vi "create.algo.watchlist.vi"(11 "Watchlist":T1[](array[typedef]) {"max.bid" format="%.2f"; "min.ask" format="%.2f"}) -> (3 "Memory.Config.Flattened":u64[](array[numeric]) format="%.0x")   [LabVIEW 2020]
uses:
  types/val.algo.pretty.watchlist.ctl
panel:
  out "Memory.Config":u64[][](array[numeric]) format="%.0x"
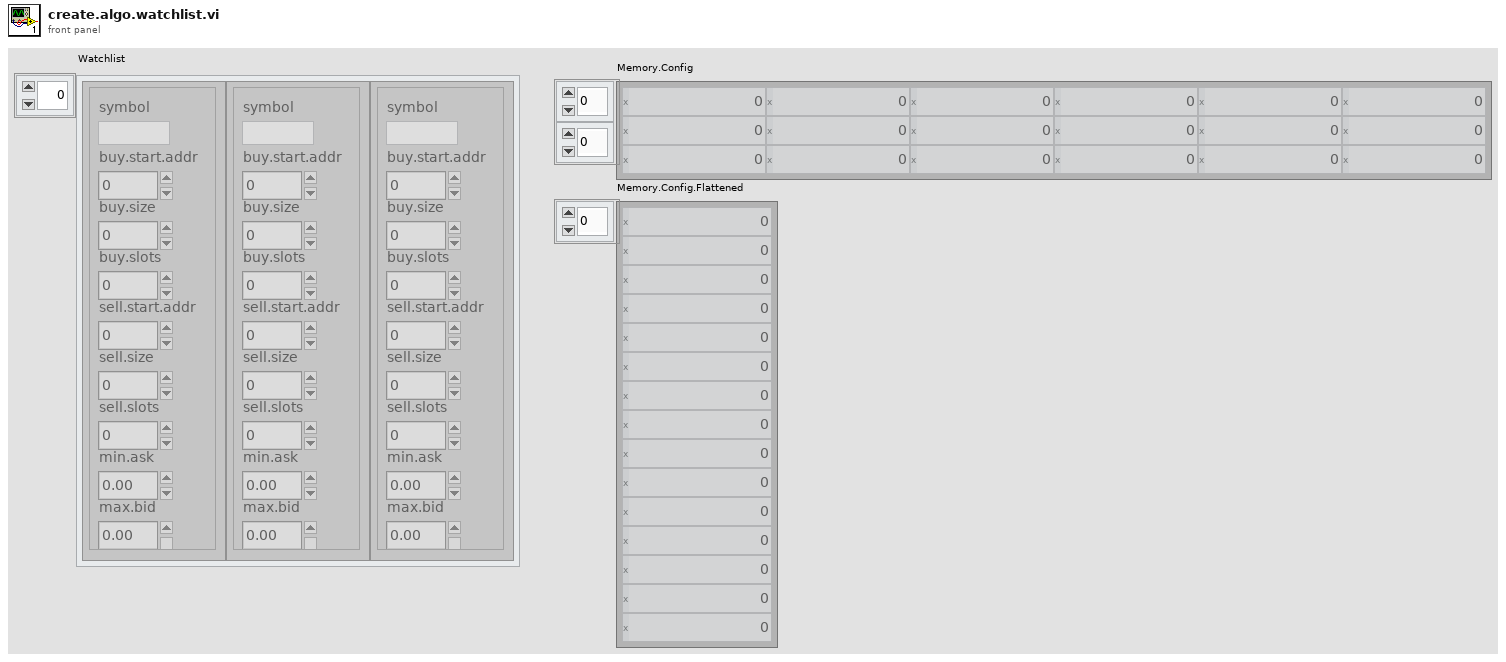
[diagram p1: front panel]
types:
  T1 = typedef "val.algo.pretty.watchlist.ctl" = cluster{"symbol":string, "buy.start.addr":u16, "buy.size":u16, "buy.slots":u16, "sell.start.addr":u16, "sell.size":u16, "sell.slots":u16, "min.ask":dbl, "max.bid":dbl}
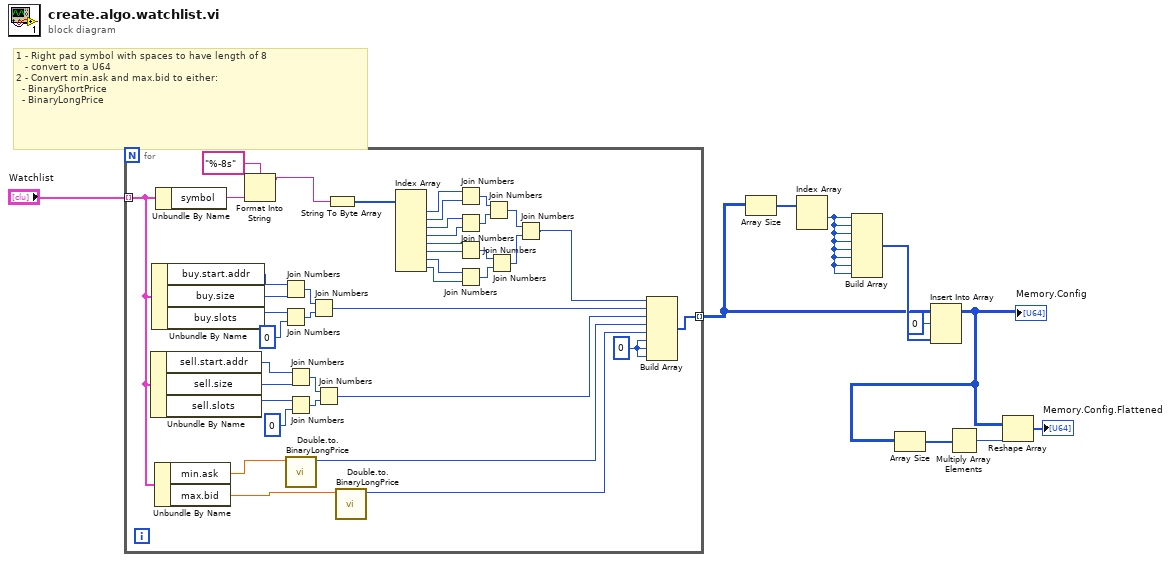
[diagram p0: block diagram]
diagram:
  # "1 - Right pad symbol with spaces to have length of 8\n   - convert to a U64\n2 - Convert min.ask and max.bid to either:\n  - BinaryShortPrice\n  - BinaryLongPrice"
  n1 = for {
    tunnel: "Watchlist" -> [w32] mode=indexing
    tunnel: [w25] -> w3 mode=indexing
    w11 = u64 0 ("element")
    n2 = Unbundle By Name(w32) -> ("sell.start.addr"=w13:u16, "sell.size"=w14:u16, "sell.slots"=w15:u16)
    n3 = Unbundle By Name(w32) -> ("buy.start.addr"=w30:u16, "buy.size"=w31:u16, "buy.slots"=w20:u16)
    n4 = Unbundle By Name(w32) -> ("min.ask"=w22:dbl, "max.bid"=w24:dbl)
    n5 = Unbundle By Name(w32) -> ("symbol"=w49:string)
    n6 = Format Into String(format string="%-8s", w49) -> (resulting string=w48:string)  [unwired: 2 in, 1 out]
    n7 = Join Numbers(hi=w30, lo=w31) -> ((hi.lo)=w29:u32)
    n8 = Join Numbers(hi=w20, lo=u16 0) -> ((hi.lo)=w28:u32)
    n9 = Join Numbers(hi=w13, lo=w14) -> ((hi.lo)=w18:u32)
    n10 = Join Numbers(hi=w15, lo=u16 0) -> ((hi.lo)=w17:u32)
    n11 = call "Double.to.BinaryLongPrice.vi"("Double"=w22) -> ("BinaryLongPrice"=w21:u64)  [unwired: 10 in]
    n12 = Join Numbers(hi=w29, lo=w28) -> ((hi.lo)=w26:u64)
    n13 = Join Numbers(hi=w18, lo=w17) -> ((hi.lo)=w12:u64)
    n14 = String To Byte Array(string=w48) -> (unsigned byte array=w33:u8[])
    n15 = call "Double.to.BinaryLongPrice.vi"("Double"=w24) -> ("BinaryLongPrice"=w23:u64)  [unwired: 10 in]
    n16 = Index Array(array=w33) -> (element #1=w47:u8, element #2=w46:u8, element #3=w45:u8, element #4=w44:u8, element #5=w43:u8, element #6=w42:u8, element #7=w41:u8, element #8=w40:u8)  [unwired: 8 in]
    n17 = Join Numbers(hi=w47, lo=w46) -> ((hi.lo)=w39:u16)
    n18 = Join Numbers(hi=w45, lo=w44) -> ((hi.lo)=w38:u16)
    n19 = Join Numbers(hi=w43, lo=w42) -> ((hi.lo)=w37:u16)
    n20 = Join Numbers(hi=w41, lo=w40) -> ((hi.lo)=w36:u16)
    n21 = Join Numbers(hi=w39, lo=w38) -> ((hi.lo)=w35:u32)
    n22 = Join Numbers(hi=w37, lo=w36) -> ((hi.lo)=w34:u32)
    n23 = Join Numbers(hi=w35, lo=w34) -> ((hi.lo)=w27:u64)
    n24 = Build Array(w27, w26, w12, w21, w23, w11, w11, w11) -> (w25:u64[])
  }
  n25 = Array Size(array=w3) -> (size(s)=w9:i32[])
  n26 = Index Array(array=w9) -> (element #1=w1:i32)  [unwired: 2 in, 1 out]
  n27 = Build Array(w1, w1, w1, w1, w1, w1, w1, w1) -> (w8:i32[])
  n28 = Insert Into Array(array=w3, index (row)=0, new element=w8) -> (w2:u64[][])  [unwired: 1 in]
  "Memory.Config" <- w2
  n29 = Array Size(array=w2) -> (size(s)=w5:i32[])
  n30 = Multiply Array Elements(1:w5) -> (0:w4:i32)
  n31 = Reshape Array(w2, w4) -> (→"Memory.Config.Flattened":u64[])
